vi "Page_Info_Validate_Filename.vi"(8 "error in (no error)":errorcluster, 10 "Filename in":string, 11 "AB_InteropAssembly in":refnum<class "AB_InteropAssembly.lvclass">) -> (0 "error out":errorcluster, 1 "hasInvalidCharacters":bool, 2 "Filename out":string, 3 "AB_InteropAssembly out":refnum<class "AB_InteropAssembly.lvclass">, 5 "message":string)   [LabVIEW 2020, in "AB_InteropAssembly.lvclass"]
uses:
  <vilib>/AppBuilder/AB_Classes/InteropAssembly/AB_InteropAssembly.lvclass
  <vilib>/AppBuilder/AB_Classes/Application/AB_Application.lvclass
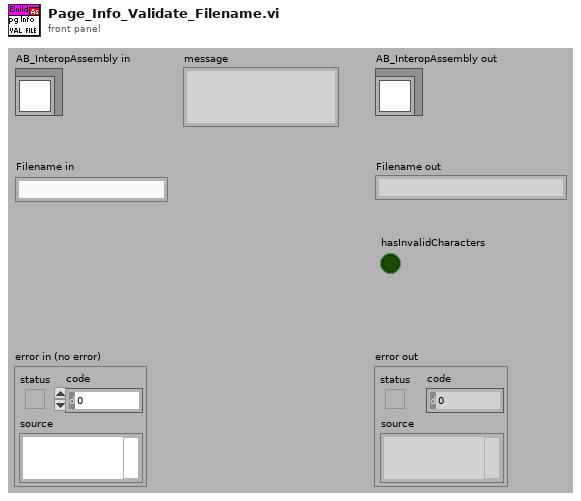
[diagram p1: front panel]
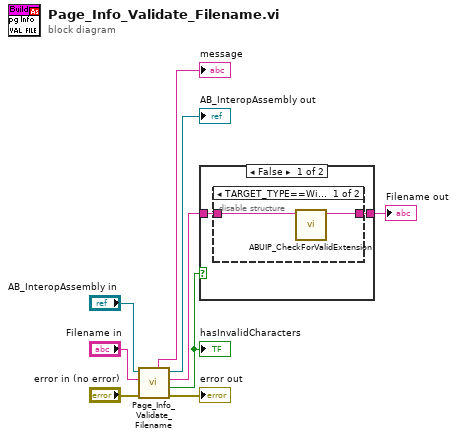
[diagram p0: block diagram]
diagram:
  n1 = call-parent "Page_Info_Validate_Filename.vi"("error in (no error)"="error in (no error)", "Filename in"="Filename in", "AB_Targetfile in"="AB_InteropAssembly in") -> ("error out"=→"error out":errorcluster, "hasInvalidCharacters"=w1:bool, "Filename out"=w3:string, "AB_Targetfile out"=→"AB_InteropAssembly out":refnum<class "AB_InteropAssembly.lvclass">, "message"=→"message":string)  [unwired: 4 out]
  "hasInvalidCharacters" <- w1
  n2 = case shown="False" w1 {
    tunnel: [w10 w15] -> w2
    tunnel: w3 -> [w11 w15]
    frame False {
      n3 = disable-structure shown="TARGET_TYPE==Windows" {
        disable-tunnel: w11 -> [w13 w14]
        disable-tunnel: [w12 w14] -> w10
        frame condition #0 (active) {
          n4 = call <resource>:"ABUIP_CheckForValidExtension.vi"("Filename in"=w13) -> ("Filename out"=w12:string)  [unwired: 10 out]
        }
        frame condition #1 {
        }
      }
    }
    frame True {
    }
  }
  "Filename out" <- w2
